vi "Pasos_por_Vuelta.vi"(4 "Tolerance":dbl, 7 "Directorio scripts ArduinoStepper.py":path=path "C:/Users/franjas/Documents/rutinas-calibracion-slm", 8 "Número de motor":string, 9 "Medir pasos por\nvuelta":bool, 10 "Minimo":dbl, 11 "Valor actual":dbl) -> (3 "Media vuelta":i32, 5 "Proceso en \nejecución":bool, 6 "Terminal output":string[](array[string]))   [LabVIEW 2013]
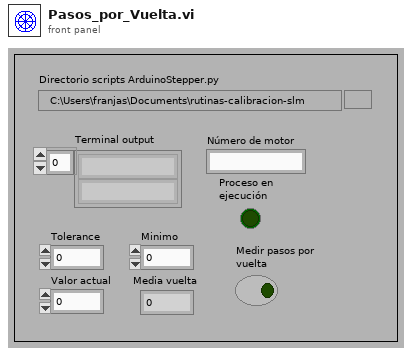
[diagram p1: front panel]
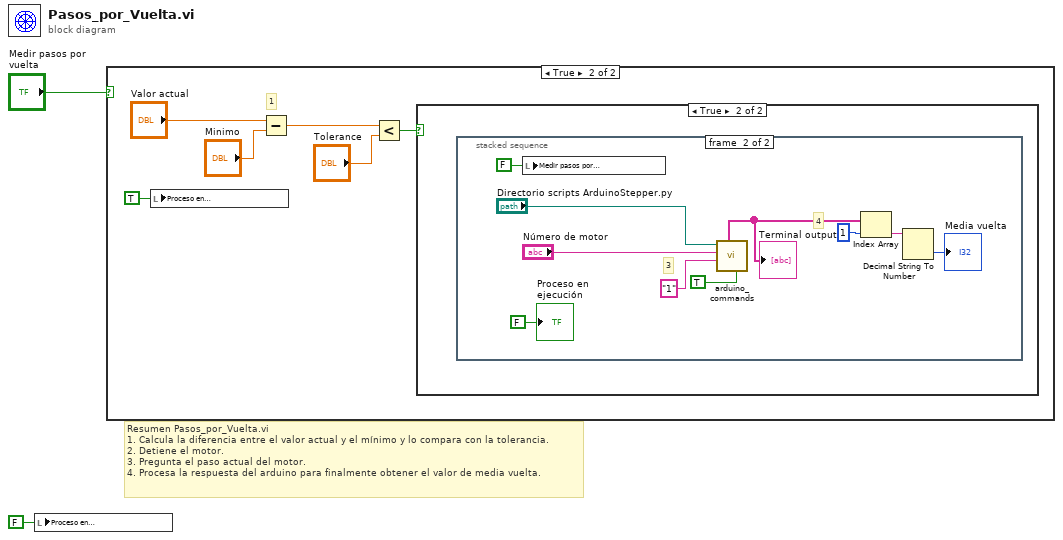
[diagram p0: block diagram]
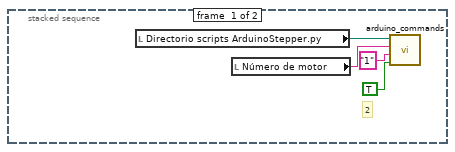
[diagram p4: hidden frame]
diagram:
  # "Resumen Pasos_por_Vuelta.vi\n1. Calcula la diferencia entre el valor actual y el mínimo y lo compara con la tolerancia.\n2. Detiene el motor.\n3. Pregunta el paso actual del motor.\n4. Procesa la respuesta del arduino para finalmente obtener el valor de media vuelta."
  n1 = local write "Proceso en \nejecución"(FALSE ("Boolean 2")) -> ()
  n2 = case shown="True" "Medir pasos por\nvuelta" {
    frame False {
    }
    frame True {
      # "1"
      n3 = local write "Proceso en \nejecución"(TRUE ("Boolean 2")) -> ()
      n4 = Subtract(x="Valor actual", y="Minimo") -> (x-y=w3:dbl)
      n5 = Less?(x=w3, y="Tolerance") -> (x < y?=w5:bool)
      n6 = case shown="True" w5 {
        frame False {
        }
        frame True {
          n7 = stacked-sequence {
            frame #0 {
              # "2"
              n8 = local read "Directorio scripts ArduinoStepper.py"() -> (w10:path)
              n9 = local read "Número de motor"() -> (w9:string)
              n10 = call "arduino_commands.vi"("Stop"=TRUE ("Constant speed"), "Argumento"="1", "Número de motor"=w9, "Directorio scripts ArduinoStepper.py"=w10) -> ()  [unwired: 7 in, 1 out]
            }
            frame #1 {
              # "4"
              # "3"
              n11 = local write "Medir pasos por\nvuelta"(FALSE ("Número de \npasos por\nvuelta")) -> ()
              n12 = call "arduino_commands.vi"("Current Step"=TRUE ("Constant speed"), "Argumento"="1", "Número de motor"="Número de motor", "Directorio scripts ArduinoStepper.py"="Directorio scripts ArduinoStepper.py") -> ("Retorno terminal"=w15:string[])  [unwired: 7 in]
              "Terminal output" <- w15
              n13 = Index Array(array=w15, index=1) -> (element=w16:string)
              n14 = Decimal String To Number(string=w16) -> (number=→"Media vuelta":i32)  [unwired: 2 in, 1 out]
              "Proceso en \nejecución" <- FALSE ("Boolean 2")
            }
          }
        }
      }
    }
  }
